vi "Gergberg Saxton.vi"() -> ()   [LabVIEW 2012, in "LightPipes.lvlib"]
uses:
  LightPipes.lvlib
panel:
  out "Waveform Graph":dbl[](graph)
  in  "Show Intensity Iterations":bool=TRUE
  in  "Show Phase Iterations":bool=TRUE
  in  "Target Phase":path=path "C:/Users/Green Beret/Documents/Visual Studio 2012/Projects/LightPipes/LightPipes/lp12src/LabView/images/phase_target.gpl"
  out "Target Phase Graph":dbl[][](graph)
  in  "size_grid":dbl=0.02
  in  "n_grid":i32=256
  in  "Source":path=path "C:/Users/Green Beret/Documents/Visual Studio 2012/Projects/LightPipes/LightPipes/lp12src/LabView/images/original/source.gpl"
  in  "Target":path=path "C:/Users/Green Beret/Documents/Visual Studio 2012/Projects/LightPipes/LightPipes/lp12src/LabView/images/original/target.gpl"
  in  "Number of Iteration":i32=10
  out "Iteration":i32=9
  out "Retrieved Target \nPhase Graph":dbl[][](graph)
  in  "Target Retrieved \nPhase":path=path "C:/Users/Green Beret/Documents/Visual Studio 2012/Projects/LightPipes/LightPipes/lp12src/LabView/images/target_retrieved_phase.gpl"
  in  "PGM gamma":dbl=1.0
  in  "forward distance":dbl=0.5
  # "Original"
  # "Target"
  # "C (forwarded from beam 1)"
  # "D (Filtered from C)"
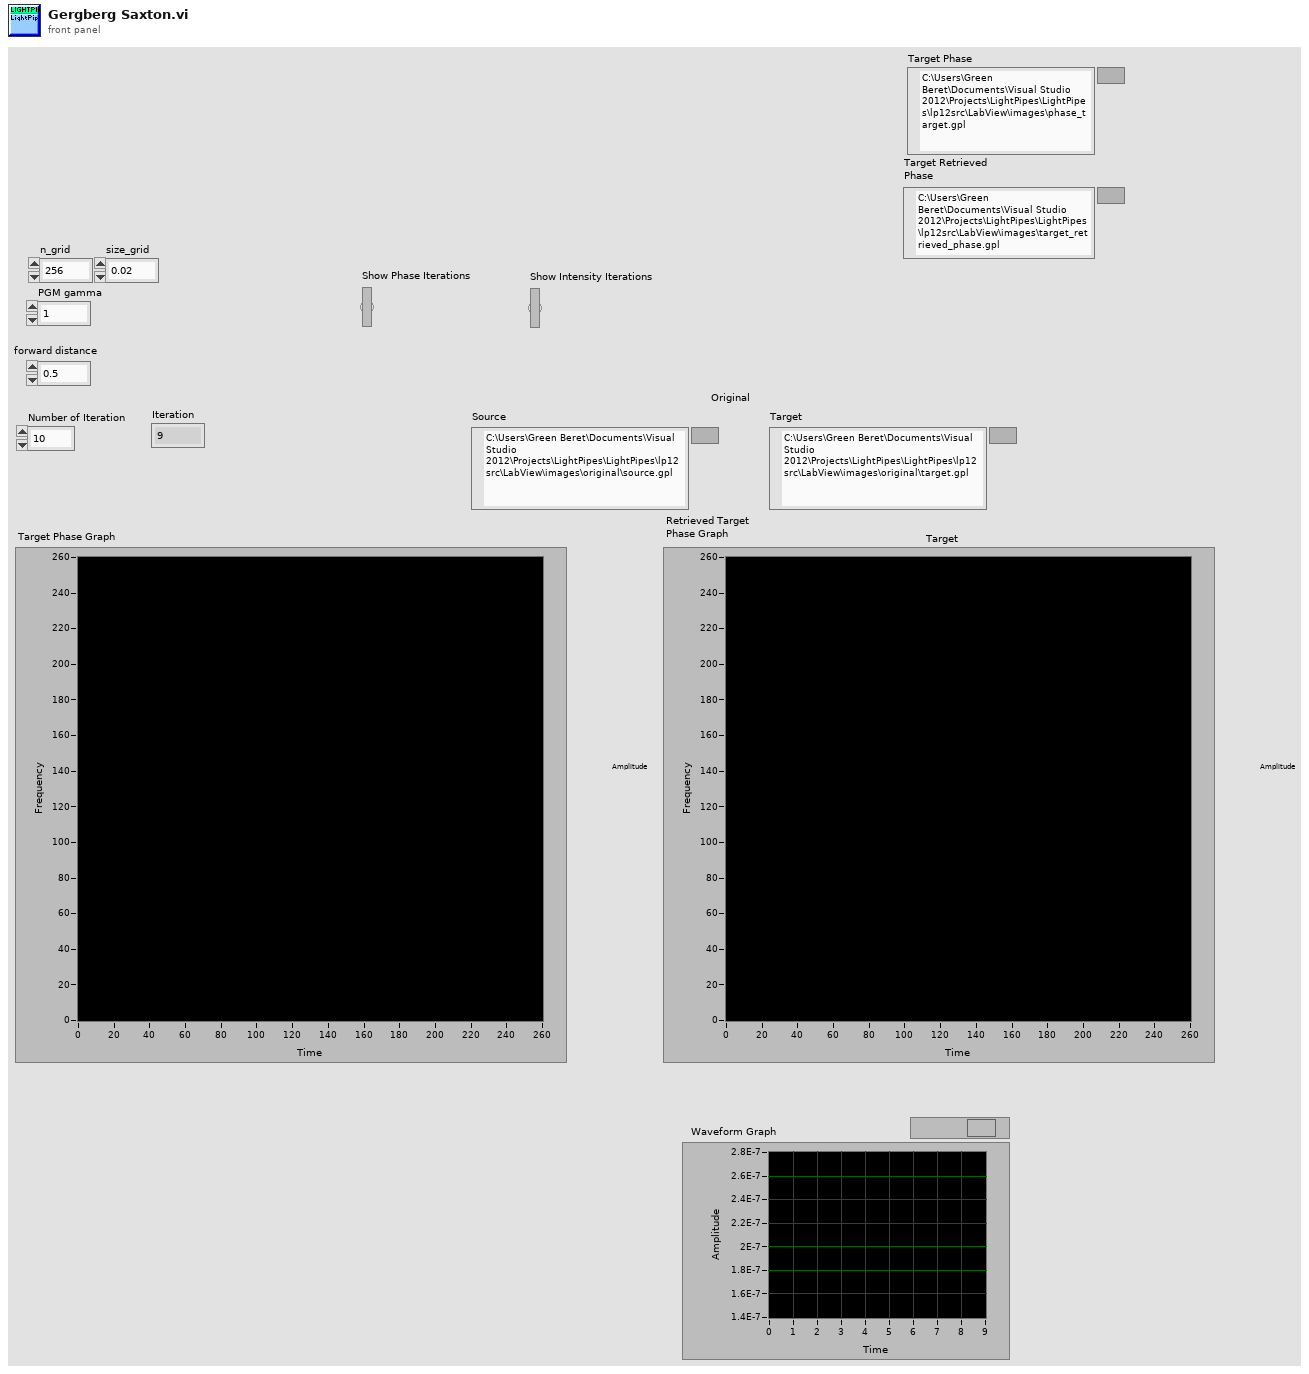
[diagram p1: front panel]
types:
  T1 = cluster{"n_grid":i32, "@dummy control@":i8, "@dummy control@":i8, "@dummy control@":i8, "@dummy control@":i8, "size":dbl, "lambda":dbl, "int1":i32, "int2":i32, "int3":i32, "@dummy control@":i8, "@dummy control@":i8, "@dummy control@":i8, "@dummy control@":i8, "double1":dbl, "double2":dbl, "double3":dbl, "real":u32, "imaginary":u32}
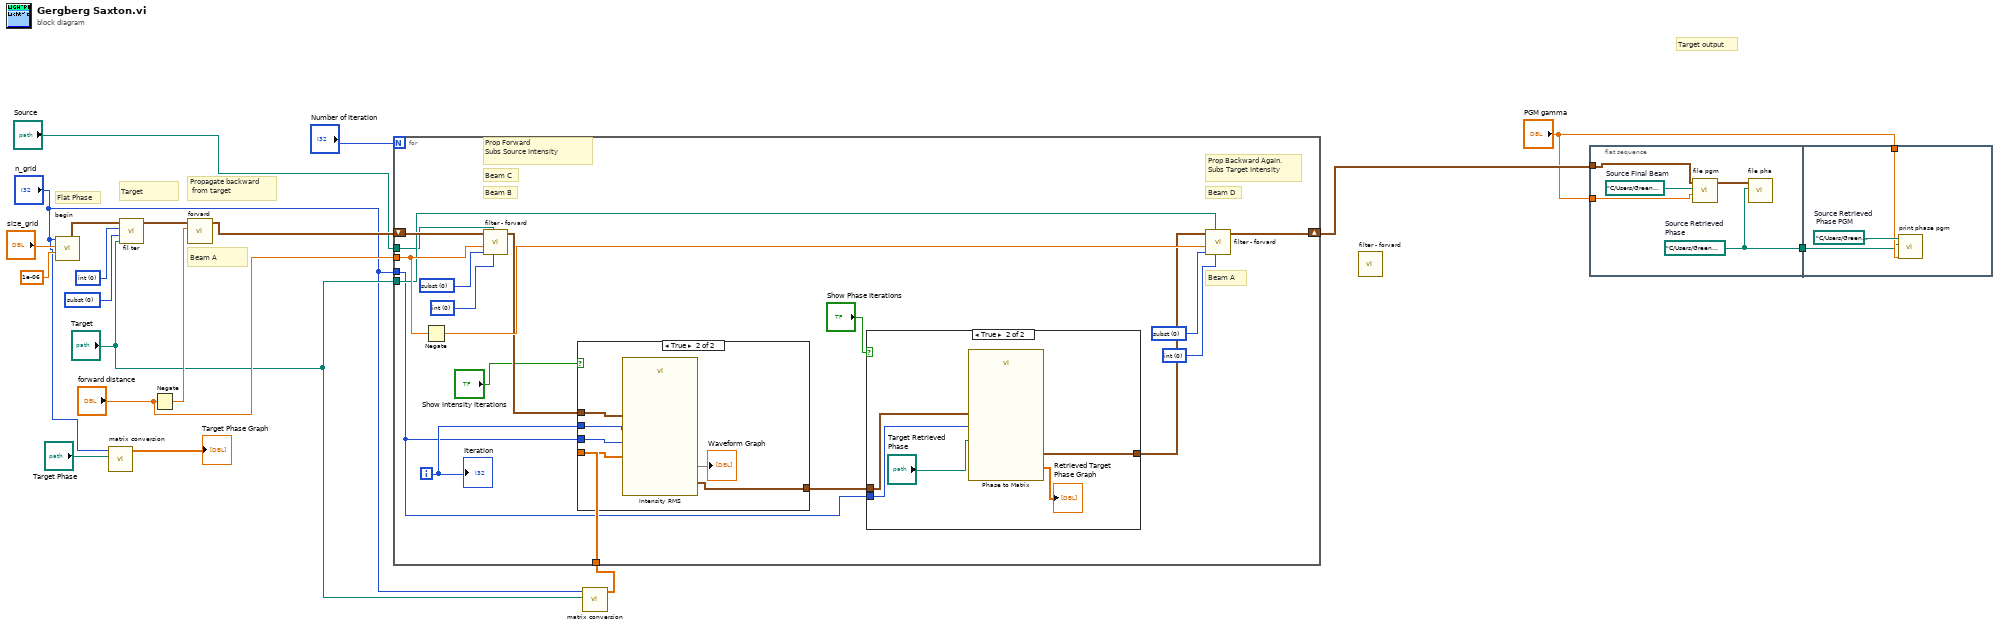
[diagram p0: block diagram]
diagram:
  w16 = i16 0 items=["subst", "mult"] ("multiplication/ substitution")
  w17 = i16 0 items=["int", "pha"] ("intensity / phase")
  # "Target output"
  # "Beam A"
  # "Target"
  # "Propagate backward\n from target"
  # "Flat Phase"
  n1 = call "begin.vi"("lambda"=1e-06, "size_grid"="size_grid", "n_grid"="n_grid") -> ("field out"=w14:T1)  [unwired: 8 in]
  n2 = call "matrix conversion.vi"("File Path"="Target Phase", "number of rows (all:-1)"="n_grid") -> ("all rows"=→"Target Phase Graph":dbl[][])  [unwired: 9 in]
  n3 = call "fil ter.vi"("Path"="Target", "multiplication/ substitution"=w16, "intensity / phase"=w17, "field"=w14) -> ("field out"=w13:T1)  [unwired: 6 in, 1 out]
  n4 = Negate(x="forward distance") -> (-x=w8:dbl)
  n5 = call "forvard.vi"("distance"=w8, "field"=w13) -> ("field out"=w11:T1)  [unwired: 9 in]
  n6 = call "matrix conversion.vi"("File Path"="Target", "number of rows (all:-1)"="n_grid") -> ("all rows"=w4:dbl[][])  [unwired: 9 in]
  n7 = for {
    N: "Number of Iteration" -> [_]
    shift-right: [w34] -> w15
    shift-left: w11 -> [w35]
    tunnel: "Target" -> [w27]
    tunnel: "forward distance" -> [w31]
    tunnel: "Source" -> [w20]
    tunnel: "n_grid" -> [w21]
    tunnel: w4 -> [w24]
    i -> [w23]
    w32 = i16 0 items=["int", "pha"] ("intensity/phase")
    w33 = i16 0 items=["subst", "mult"] ("multiplication/substitution")
    w36 = i16 0 items=["int", "pha"] ("intensity/phase")
    w37 = i16 0 items=["subst", "mult"] ("multiplication/substitution")
    # "Beam A"
    # "Beam D"
    # "Beam C"
    # "Beam B"
    # "Prop Backward Again.\nSubs Target Intensity"
    # "Prop Forward\nSubs Source Intensity"
    n8 = Negate(x=w31) -> (-x=w30:dbl)
    n9 = call "filter - forvard .vi"("intensity/phase"=w36, "path filter in"=w20, "multiplication/substitution"=w37, "forward distance"=w31, "field"=w35) -> ("field out"=w26:T1)  [unwired: 3 in, 2 out]
    n10 = case shown="True" "Show Intensity Iterations" {
      tunnel: w26 -> [w38 w44]
      tunnel: [w38 w43] -> w25
      tunnel: w24 -> [_ w41]
      tunnel: w23 -> [_ w40]
      tunnel: w21 -> [_ w39]
      frame False {
      }
      frame True {
        n11 = call "Intensity RMS.vi"("Original Intensity"=w41, 9:w40, "num rows"=w39, "field"=w44) -> (2:→"Waveform Graph", "field out"=w43:T1)  [unwired: 5 in, 1 out]
      }
    }
    n12 = case shown="True" "Show Phase Iterations" {
      tunnel: w25 -> [w45 w49]
      tunnel: [w45 w50] -> w29
      tunnel: w21 -> [_ w48]
      frame False {
      }
      frame True {
        n13 = call "Phase to Matrix.vi"("Target Retrieved \nPhase"="Target Retrieved \nPhase", "num rows"=w48, "field"=w49) -> ("Phase"=→"Retrieved Target \nPhase Graph":dbl[][], "field out"=w50:T1)  [unwired: 7 in]
      }
    }
    n14 = call "filter - forvard .vi"("intensity/phase"=w32, "path filter in"=w27, "multiplication/substitution"=w33, "forward distance"=w30, "field"=w29) -> ("field out"=w34:T1)  [unwired: 3 in, 2 out]
    "Iteration" <- w23
  }
  n15 = call "filter - forvard .vi"() -> ()  [unwired: 8 in, 3 out]
  n16 = flat-sequence {
    tunnel: w15 -> [w55]
    tunnel: "PGM gamma" -> [w53]
    tunnel: [w51] -> w19
    tunnel: "PGM gamma" -> [w57]
    tunnel: w19 -> [w56]
    frame #0 {
      w51 = path "C:/Users/Green Beret/Documents/Visual Studio 2012/Projects/LightPipes/LightPipes/lp12src/LabView/images/source_retrieved_phase.gpl"  # Source Retrieved  Phase
      w54 = path "C:/Users/Green Beret/Documents/Visual Studio 2012/Projects/LightPipes/LightPipes/lp12src/LabView/images/source_final.pgm"  # Source Final Beam
      n17 = call "file pgm.vi"("gamma"=w53, "Path"=w54, "field"=w55) -> ("field out"=w52:T1)  [unwired: 7 in, 1 out]
      n18 = call "file pha.vi"("Path in"=w51, "field"=w52) -> ()  [unwired: 8 in, 2 out]
    }
    frame #1 {
      w58 = path "C:/Users/Green Beret/Documents/Visual Studio 2012/Projects/LightPipes/LightPipes/lp12src/LabView/images/source_retrieved_phase.pgm"  # Source Retrieved  Phase PGM
      n19 = call "print phase pgm.vi"("gamma"=w57, "Source Phase"=w56, "Source Phase PGM"=w58) -> ()  [unwired: 9 in]
    }
  }
